vi "Facade.vi"(0 "Data In":T5, 2 "Display State In":T3, 3 "Container State":T4) -> (6 "Data Out":T5, 7 "Display State Out":T3, 8 "Action":T2)   [LabVIEW 2015, in "Digital I-O.xctl"]
uses:
  Digital I-O.xctl
  Data.ctl
  <vilib>/_xctls/Container State.ctl
  State.ctl
  <vilib>/_xctls/Action.ctl
  <vilib>/_xctls/XControlSupport.lvlib
panel:
  in  "DIO":T1 caption="Slot X"
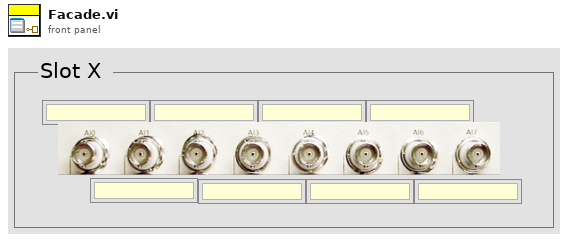
[diagram p1: front panel]
types:
  T1 = cluster{"DIO0":u16, "DIO1":u16, "DIO2":u16, "DIO3":u16, "DIO4":u16, "DIO5":u16, "DIO6":u16, "DIO7":u16}
  T2 = typedef "XControlSupport.lvlib/Action.ctl" = cluster{"Data Changed?":bool, "State Changed?":bool, "Action Name":string}
  T3 = typedef "Digital I-O.xctl/State.ctl" = cluster{"Hide unused":bool, "Is dirty?":bool, "SlotNum":i32, "Output List":string[], "Input List":string[]}
  T4 = typedef "XControlSupport.lvlib/Container State.ctl" = cluster{"Indicator?":bool, "Run Mode?":bool, " Refnum":refnum<vi>}
  T5 = typedef "Digital I-O.xctl/Data.ctl" = cluster{"Connections":string[]}
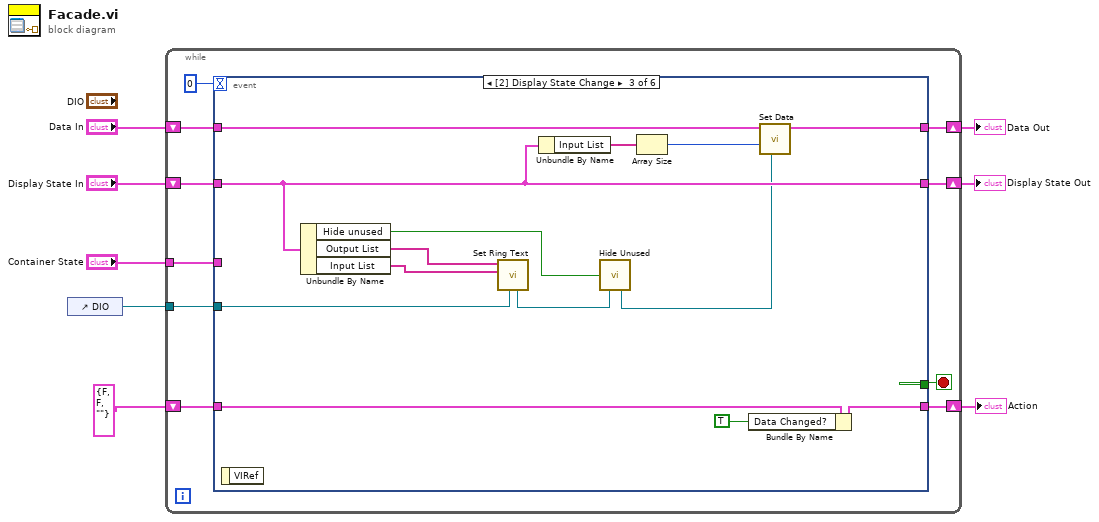
[diagram p0: block diagram]
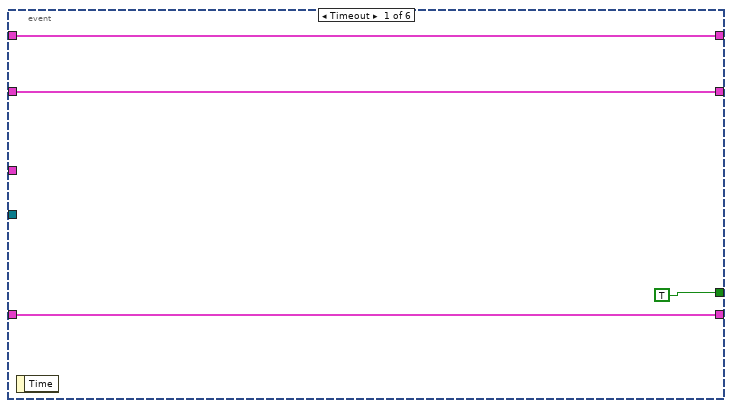
[diagram p2: hidden frame]
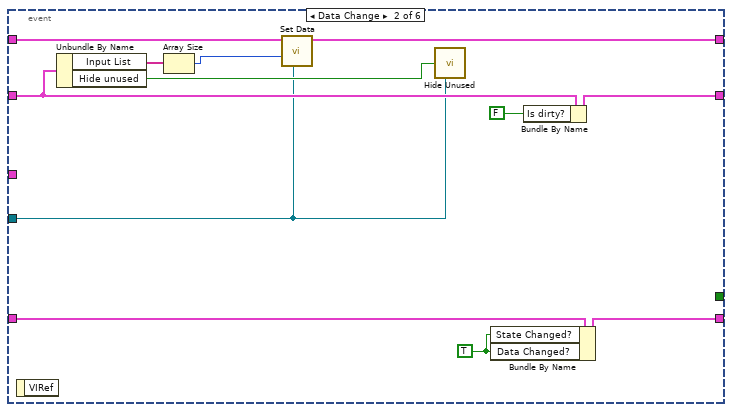
[diagram p3: hidden frame]
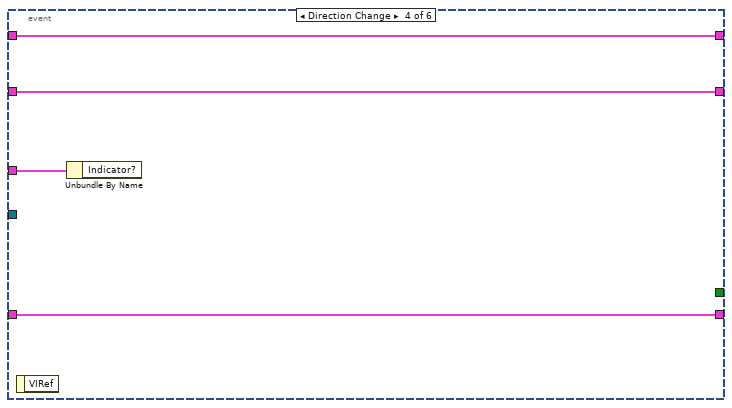
[diagram p4: hidden frame]
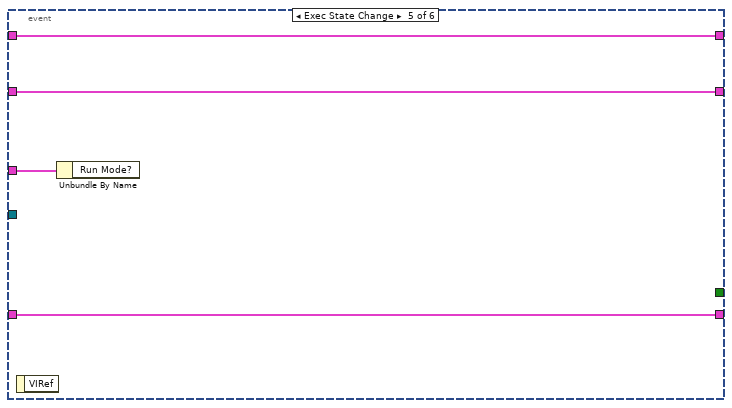
[diagram p5: hidden frame]
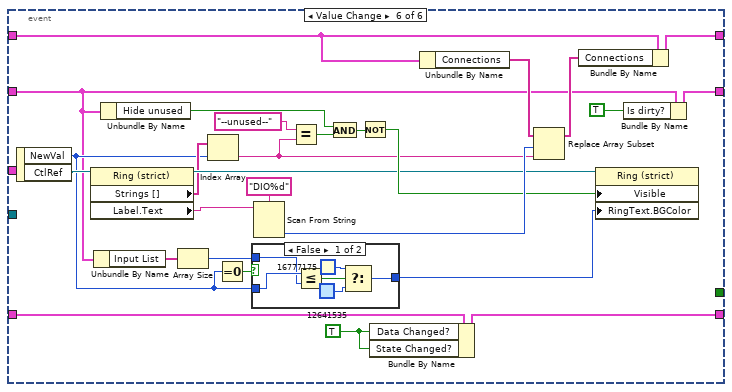
[diagram p6: hidden frame]
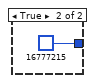
[diagram p7: hidden frame]
diagram:
  n1 = control-ref of="DIO"() -> (w1:refnum<vi>)
  n2 = while {
    shift-right: [w17] -> w5
    shift-left: "Display State In" -> [w18]
    tunnel: "Container State" -> [w14]
    shift-right: [w12] -> w8
    shift-left: "Data In" -> [w13]
    shift-right: [w10] -> w3
    shift-left: T2 {"Data Changed?"=FALSE, "State Changed?"=FALSE, "Action Name"=""} ("Action") -> [w11]
    tunnel: w1 -> [w9]
    stop <- w16 stop-if-true
    n3 = event shown="[2] Display State Change" {
      selector: _ -> [_ _ _ _ _ _]
      dyn-events: _ -> [_ _ _ _ _ _]
      timeout: 0 -> [_ _ _ _ _ _]
      tunnel: w18 -> [w20 w29 w39 w51 w55 w60]
      tunnel: [w20 w27 w39 w51 w55 w68] -> w17
      tunnel: [TRUE _ _ _ _ _] -> w16
      tunnel: w14 -> [_ _ _ w52 w56 _]
      tunnel: w13 -> [w19 w34 w45 w50 w54 w82]
      tunnel: [w19 w33 w44 w50 w54 w80] -> w12
      tunnel: [w21 w31 w46 w49 w53 w78] -> w10
      tunnel: w11 -> [w21 w32 w47 w49 w53 w79]
      tunnel: w9 -> [_ w25 w40 _ _ _]
      event Timeout {
        n4 = event-data() -> ()  [unwired: 1 in, 1 out]
      }
      event Data Change {
        w30 = TRUE ("Data Changed?")
        n5 = event-data() -> ()  [unwired: 1 in, 1 out]
        n6 = Unbundle By Name(w29) -> ("Input List"=w24:string[], "Hide unused"=w26:bool)
        n7 = Array Size(array=w24) -> (size(s)=w23:i32)
        n8 = call "Set Data.vi"("DIO ref"=w25, "NInput"=w23, "Data"=w34) -> ("Data out"=w33:T5)  [unwired: 8 in]
        n9 = call "Hide Unused.vi"("Hide unused"=w26, "DIO ref"=w25) -> ()  [unwired: 13 in, 1 out]
        n10 = Bundle By Name(cluster=w32, "State Changed?"=w30, "Data Changed?"=w30) -> (w31:T2)
        n11 = Bundle By Name(cluster=w29, "Is dirty?"=FALSE) -> (w27:T3)
      }
      event Display State Change {
        n12 = event-data() -> ()  [unwired: 1 in, 1 out]
        n13 = Unbundle By Name(w39) -> ("Hide unused"=w48:bool, "Output List"=w43:string[], "Input List"=w42:string[])
        n14 = call "Set Ring Text.vi"("DIO ref"=w40, "Inputs"=w42, "Outputs"=w43) -> ("DIO ref out"=w35:refnum<vi>)  [unwired: 8 in]
        n15 = Unbundle By Name(w39) -> ("Input List"=w38:string[])
        n16 = call "Hide Unused.vi"("Hide unused"=w48, "DIO ref"=w35) -> ("DIO ref out"=w36:refnum<vi>)  [unwired: 13 in]
        n17 = Array Size(array=w38) -> (size(s)=w37:i32)
        n18 = Bundle By Name(cluster=w47, "Data Changed?"=TRUE) -> (w46:T2)
        n19 = call "Set Data.vi"("DIO ref"=w36, "NInput"=w37, "Data"=w45) -> ("Data out"=w44:T5)  [unwired: 8 in]
      }
      event Direction Change {
        n20 = event-data() -> ()  [unwired: 1 in, 1 out]
        n21 = Unbundle By Name(w52) -> ()  [unwired: 1 out]
      }
      event Exec State Change {
        n22 = event-data() -> ()  [unwired: 1 in, 1 out]
        n23 = Unbundle By Name(w56) -> ()  [unwired: 1 out]
      }
      event "DIO.DIO0", "DIO.DIO1", "DIO.DIO2", "DIO.DIO3", "DIO.DIO4", "DIO.DIO5", "DIO.DIO6", "DIO.DIO7": Value Change {
        w70 = TRUE ("Data Changed?")
        n24 = event-data() -> ("NewVal"=w61:u16, "CtlRef"=w73:refnum<vi>)  [unwired: 1 in]
        n25 = property class="Ring (strict)"(reference=w73) -> (reference out=w64:refnum<vi>, "Strings []"=w63:string[], "Label.Text"=w65:string)  [unwired: 1 in, 1 out]
        n26 = Unbundle By Name(w60) -> ("Input List"=w59:string[])
        n27 = Unbundle By Name(w60) -> ("Hide unused"=w74:bool)
        n28 = Array Size(array=w59) -> (size(s)=w58:i32)
        n29 = Index Array(array=w63, index=w61) -> (element=w67:string)
        n30 = Equal To 0?(x=w61) -> (x = 0?=w62:bool)
        n31 = case shown="False" w62 {
          tunnel: w61 -> [w89 _]
          tunnel: w58 -> [w88 _]
          tunnel: [w84 u32 16777215] -> w57
          frame False {
            n32 = Less Or Equal?(x=w89, y=w88) -> (x <= y?=w87:bool)
            n33 = Select(t=u32 16777175, s=w87, f=u32 12641535) -> (s? t:f=w84:u32)
          }
          frame True {
          }
        }
        n34 = Scan From String(format string="DIO%d", input string=w65) -> (output 1=w76:i32)  [unwired: 3 in, 3 out]
        n35 = Equal?(x="--unused--", y=w67) -> (x = y?=w75:bool)
        n36 = And(x=w74, y=w75) -> (x .and. y?=w72:bool)
        n37 = Not(x=w72) -> (.not. x?=w71:bool)
        n38 = Bundle By Name(cluster=w79, "Data Changed?"=w70, "State Changed?"=w70) -> (w78:T2)
        n39 = Unbundle By Name(w82) -> ("Connections"=w83:string[])
        n40 = Replace Array Subset(array=w83, new element=w67, index=w76) -> (w81:string[])
        n41 = Bundle By Name(cluster=w82, "Connections"=w81) -> (w80:T5)
        n42 = property class="Ring (strict)"(reference=w64, "Visible"=w71, "RingText.BGColor"=w57) -> ()  [unwired: 1 in, 2 out]
        n43 = Bundle By Name(cluster=w60, "Is dirty?"=TRUE) -> (w68:T3)
      }
    }
  }
  "Display State Out" <- w5
  "Data Out" <- w8
  "Action" <- w3
